vi "Sweep Control Inner Loop.vi"(8 "error in (no error)":errorcluster, 9 "index":i32, 10 "loop #":i32, 11 "SweepControl in":refnum<class "SweepControl.lvclass">) -> (0 "error out":errorcluster, 2 "Stop?":bool, 3 "SweepControl out":refnum<class "SweepControl.lvclass">)   [LabVIEW 2016, in "SweepControl.lvclass"]
uses:
  SweepControl.lvclass
  SweepControl.lvclass/SweepControl.ctl
  <userlib>/_OpenG.lib/array/array.llb/Empty 1D Array (Variant)__ogtk.vi
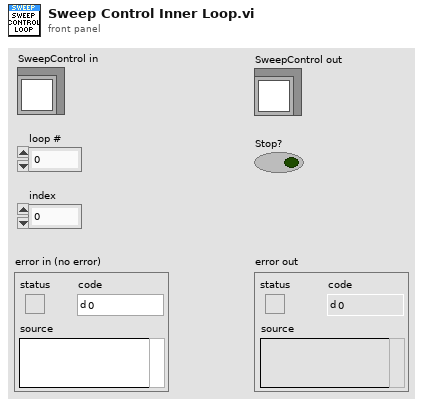
[diagram p1: front panel]
types:
  T1 = typedef "SweepControl.lvclass/ScanControl.ctl" = T2[]
  T2 = typedef "SweepControl.lvclass/Cluster - ScanControl.ctl" = cluster{"Priority":T3, "Scan name":T4}
  T3 = typedef "SweepControl.lvclass/Enum - Priority.ctl" = enum16{"Priority 0", "Priority 1", "Priority 2", "Priority 3", "Priority 4", "Priority 5"}
  T4 = typedef "SweepControl.lvclass/Enum - Action.ctl" = enum16{"OFF", "DSA_Vamp", "DSA_freq", "DSA_Vsg1", "DSA_Vsg2", "DSA_Vsg3", "DAQ_Vbg", "B_Field", "Humidity", "Temp", "MW_freq1", "MW_freq2", "MW_amplitude1", "MW_amplitude2"}
  T5 = typedef "SweepControl.lvclass/PostAction.ctl" = T6[]
  T6 = typedef "SweepControl.lvclass/Enum - PostAction.ctl" = enum16{"Clear DAQ Tasks", "Check Temperature", "Wait", "Do Nothing"}
  T7 = cluster{"Inner Loop Index":i32, "Scan Action Loop Index":i32, "loop #":i32}
  T8 = typedef "SweepControl.lvclass/Cluster - ScanParamters.ctl" = cluster{"DAQ Channel":i32, "Label":string, "Start":dbl, "End":dbl, "Step":dbl, "Rate":dbl, "VISA resource name":refnum<visa-resource-name>, "wait (ms)":u32}
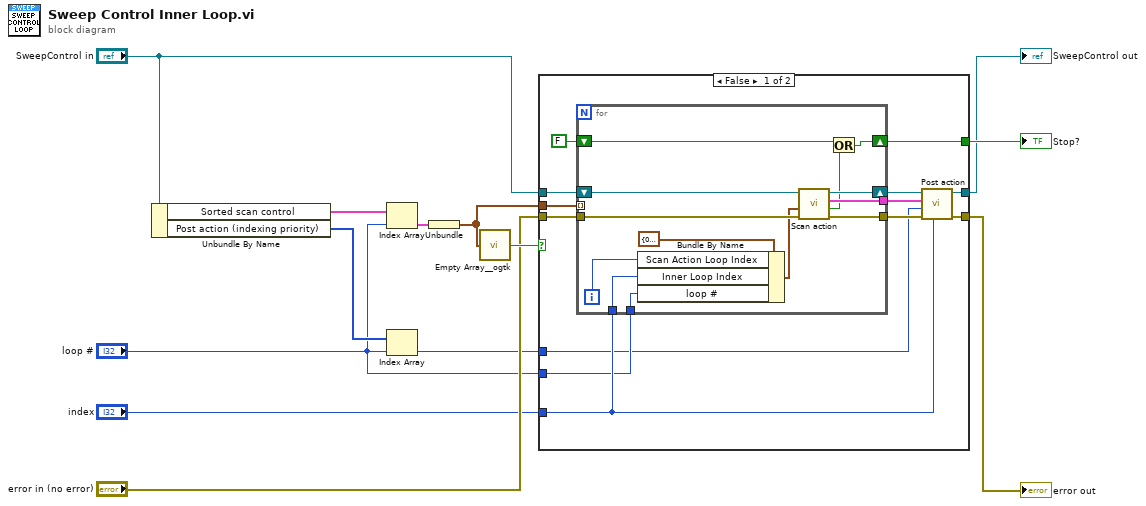
[diagram p0: block diagram]
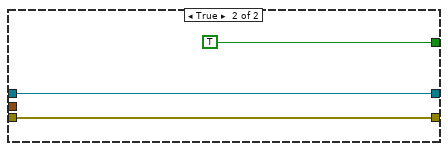
[diagram p2: hidden frame]
diagram:
  n1 = Unbundle By Name("SweepControl in") -> ("Sorted scan control"=w10:cluster{T1}[], "Post action (indexing priority)"=w9:T5)
  n2 = Index Array(array=w10, index="loop #") -> (element=w11:cluster{T1})
  n3 = Index Array(array=w9, index="loop #") -> (element=w2:T6)
  n4 = Unbundle(w11) -> (w1:T1)
  n5 = call-poly <userlib>:"Empty Array__ogtk.vi"("Array"=w1) -> ("Empty Array?"=w12:bool)  [unwired: 8 in]
  n6 = case shown="False" w12 {
    tunnel: [w24 TRUE ("Stop?")] -> w13
    tunnel: "loop #" -> [w16 _]
    tunnel: "error in (no error)" -> [w22 w40]
    tunnel: [w23 w40] -> w7
    tunnel: "index" -> [w20 _]
    tunnel: "SweepControl in" -> [w19 w39]
    tunnel: [w18 w39] -> w4
    tunnel: w2 -> [w15 _]
    tunnel: w1 -> [w14 _]
    frame False {
      n7 = for {
        shift-right: [w35] -> w24
        shift-left: FALSE -> [w38]
        tunnel: w22 -> [w37]
        tunnel: [w36] -> w21
        tunnel: w20 -> [w29]
        shift-right: [w33] -> w18
        shift-left: w19 -> [w34]
        tunnel: [w32] -> w17
        tunnel: w16 -> [w28]
        tunnel: w14 -> [_] mode=indexing
        i -> [w30]
        n8 = Bundle By Name(cluster=T7 {"Inner Loop Index"=0, "Scan Action Loop Index"=0, "loop #"=0} ("Indices"), "Scan Action Loop Index"=w30, "Inner Loop Index"=w29, "loop #"=w28) -> (w27:T7)
        n9 = call "Scan action.vi"("error in (no error)"=w37, "Indices"=w27, "SweepControl in"=w34) -> ("error out"=w36:errorcluster, "Stop?"=w31:bool, "Scan Parameters"=w32:T8, "SweepControl out"=w33:refnum<class "SweepControl.lvclass">)  [unwired: 5 in]
        n10 = Or(x=w38, y=w31) -> (x .or. y?=w35:bool)
      }
      n11 = call "Post action.vi"("Index"=w20, "error in (no error)"=w21, "PostAction"=w15, "Scan Parameters"=w17) -> ("error out"=w23:errorcluster)  [unwired: 7 in]
    }
    frame True {
    }
  }
  "SweepControl out" <- w4
  "Stop?" <- w13
  "error out" <- w7
